vi "ROI entry screen-Calculate cycle rate.vi"(8 "error in (no error)":errorcluster, 11 "Total ROI time":dbl) -> (0 "error out":errorcluster, 3 "Estimated cycle rate":dbl)   [LabVIEW 2020]
uses:
  Global Variables/General Globals.vi
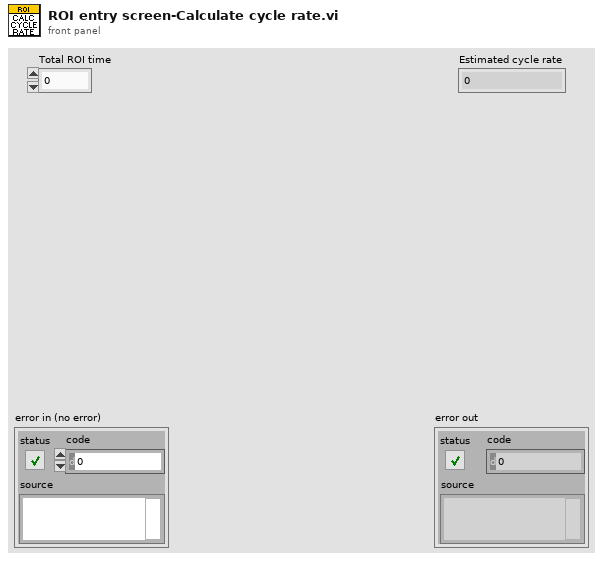
[diagram p1: front panel]
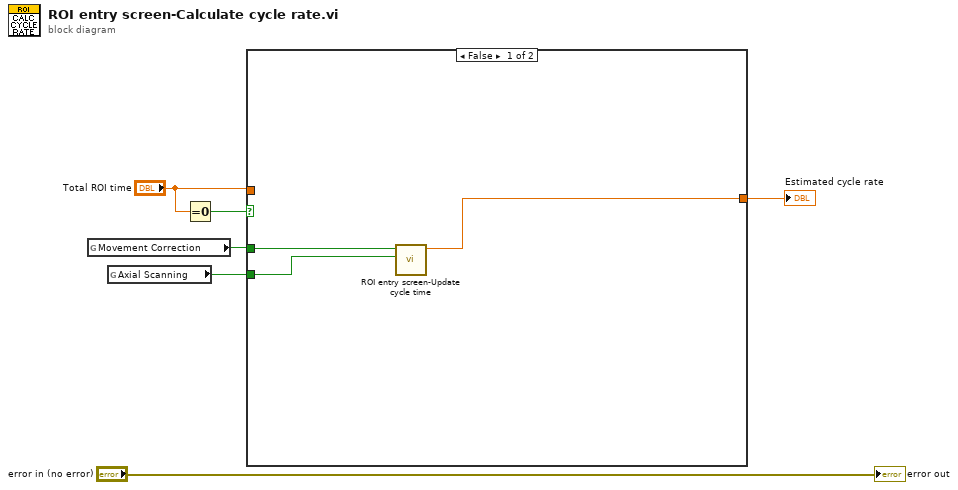
[diagram p0: block diagram]
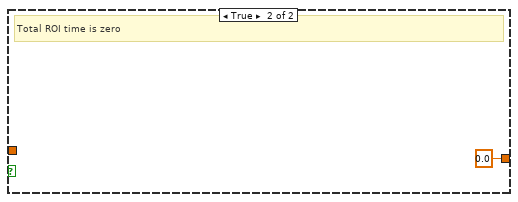
[diagram p2: hidden frame]
diagram:
  n1 = global read "General Globals.vi" "Movement Correction"() -> (w2:bool)
  n2 = global read "General Globals.vi" "Axial Scanning"() -> (w1:bool)
  n3 = Equal To 0?(x="Total ROI time") -> (x = 0?=w3:bool)
  n4 = case shown="False" w3 {
    tunnel: [w8 0.0] -> w6
    tunnel: "Total ROI time" -> [_ _]
    tunnel: w2 -> [w9 _]
    tunnel: w1 -> [w7 _]
    frame False {
      n5 = call "ROI entry screen-Update cycle time.vi"("AXIAL MC ON ?"=w7, "MC ON ?"=w9) -> ("Cycle rate (Hz)"=w8:dbl)  [unwired: 6 in, 3 out]
    }
    frame True {
      # "Total ROI time is zero"
    }
  }
  "Estimated cycle rate" <- w6
  "error out" <- "error in (no error)"
